vi "Init.vi"(7 "Variables":refnum<class "Variables.lvclass">, 8 "error in (no error)":errorcluster, 9 "Condition Config":refnum<class "Condition Config.lvclass">, 10 "VolatusAPI":refnum<class "VolatusAPI.lvclass">, 11 "Condition in":refnum<class "Condition.lvclass">) -> (0 "error out":errorcluster, 3 "Condition out":refnum<class "Condition.lvclass">)   [LabVIEW 2020]
uses:
  Condition.lvclass
  Volatus/VolatusAPI/VolatusAPI.lvclass
  Variables/Variables.lvclass
  VolatusSeqConfig/Condition Config/Condition Config.lvclass
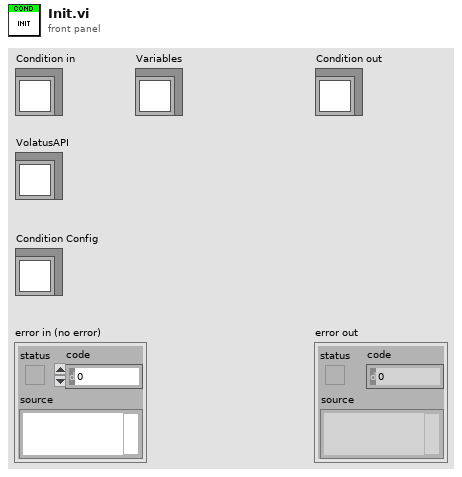
[diagram p1: front panel]
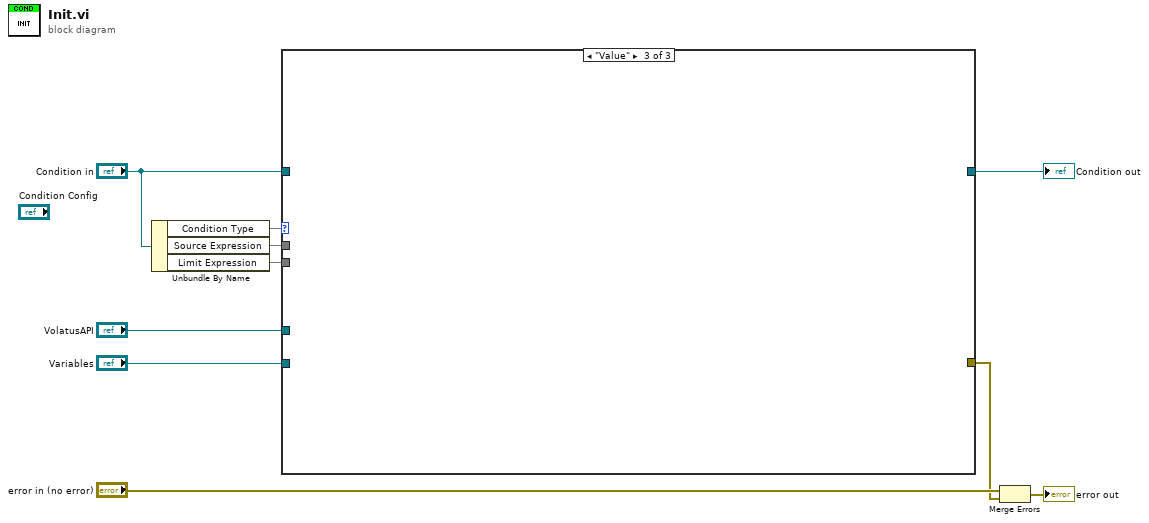
[diagram p0: block diagram]
diagram:
  n1 = Unbundle By Name("Condition in") -> ("Condition Type"=w9, "Source Expression"=w6, "Limit Expression"=w5)
  n2 = case shown="\"Value\"" w9 {
    tunnel: "Condition in" -> [w11 w12 w15]
    tunnel: [w11 w12 _] -> w7
    tunnel: w6 -> [_ _ w13]
    tunnel: w5 -> [_ _ _]
    tunnel: "VolatusAPI" -> [_ _ w14]
    tunnel: "Variables" -> [_ _ w16]
    tunnel: [_ _ _] -> w1
    frame "Immediate" {
      # "Always transitions, nothing to init."
    }
    frame "Time" {
      # "Nothing to init for time conditions"
    }
    frame "Value" {
    }
  }
  "Condition out" <- w7
  n3 = Merge Errors("error in (no error)", w1) -> (→"error out":errorcluster)
